vi "例6-1.vi"() -> ()   [LabVIEW 2019]
uses:
  <vilib>/Analysis/NI_AALBase.lvlib
panel:
  in  "采样点数":dbl=1000.0
  in  "采样频率":dbl=1000.0
  in  "初始相位":dbl
  in  "信号幅度":dbl=1.0
  in  "信号频率":dbl=5.0
  out "波形图":cluster{i32, dbl, "sine wave":dbl[]}(graph)
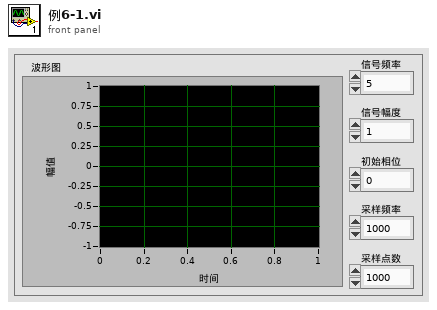
[diagram p1: front panel]
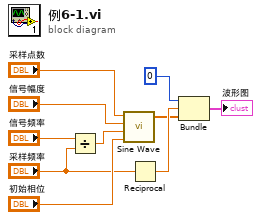
[diagram p0: block diagram]
diagram:
  n1 = Divide(x="信号频率", y="采样频率") -> (x/y=w7:dbl)
  n2 = call <vilib>:"Sine Wave.vi"("samples"="采样点数", "amplitude"="信号幅度", "frequency"=w7, "phase in"="初始相位") -> ("sine wave"=w2:dbl[])  [unwired: 1 in, 2 out]
  n3 = Reciprocal(x="采样频率") -> (1/x=w3:dbl)
  n4 = Bundle("t0"=0, w3, "sine wave"=w2) -> (→"波形图":cluster{"t0":i32, dbl, "sine wave":dbl[]})  [unwired: 1 in]
